vi "ArrayColorU32ToImage.vi"(8 "error in":errorcluster, 10 "Pixel":u32[][](array[numeric]), 11 "Image Reference In":T1) -> (0 "error out":errorcluster, 3 "Image Reference Out":T1)   [LabVIEW 2020, in "OpenLvVision_Image.lvlib" / "DataAccess.lvlib"]
doc: "Replaces the image's data with the provided array (Copy)"
uses:
  DataAccess.lvlib
  Management/TypeDef/Image.ctl
  Management/Management.lvlib
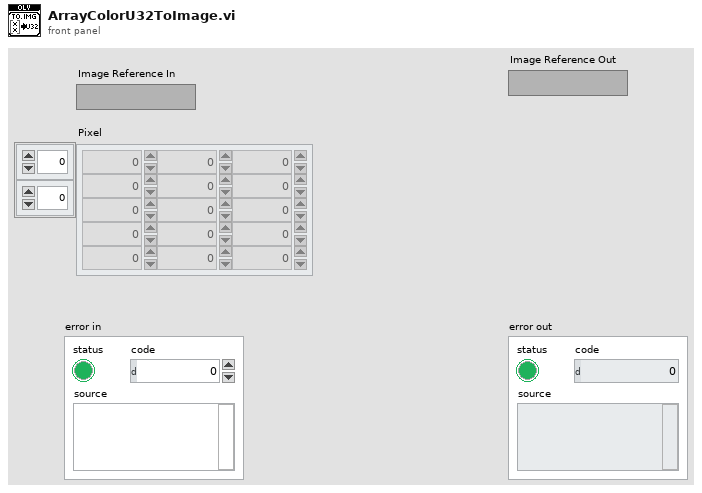
[diagram p1: front panel]
types:
  T1 = typedef "OpenLvVision_Image.lvlib/Management.lvlib/Image.ctl" = refnum<image>
  T2 = typedef "IMAQ Image.ctl" = refnum<image>
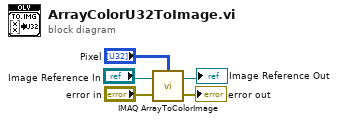
[diagram p0: block diagram]
diagram:
  n1 = call "IMAQ ArrayToColorImage"("Image Pixels (U32)"="Pixel", "Image"="Image Reference In", "error in (no error)"="error in") -> ("Image Out"=→"Image Reference Out":T2, "error out"=→"error out":errorcluster)  [unwired: 2 in]
